vi "Read Date and Time.vi"(8 "error in (no error)":errorcluster, 11 "VISA resource name":refnum<visa-resource-name>) -> (0 "error out":errorcluster, 1 "Time":string, 2 "Date":string, 3 "VISA resource name out":refnum<visa-resource-name>)   [LabVIEW 2014, in "Fluke 190 Series II.lvlib"]
doc: "Returns the date and time setting of the real time clock in the testtool."
uses:
  Fluke 190 Series II.lvlib
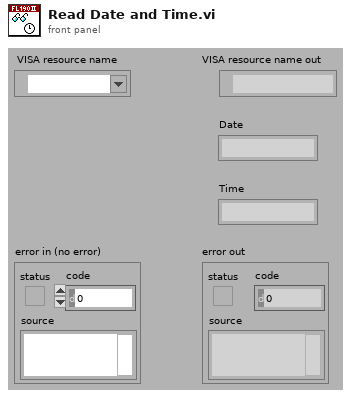
[diagram p1: front panel]
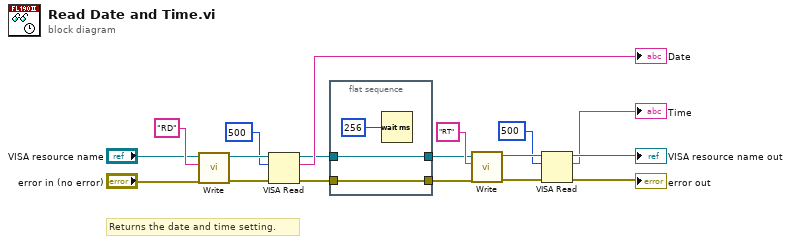
[diagram p0: block diagram]
diagram:
  # "Returns the date and time setting."
  n1 = call "Write.vi"("error in (no error)"="error in (no error)", "Write Buffer"="RD", "VISA resource name"="VISA resource name") -> ("error out"=w14:errorcluster, "VISA resource name out"=w15:refnum<visa-resource-name>)  [unwired: 7 out]
  n2 = VISA Read(VISA resource name=w15, byte count=u32 500, error in (no error)=w14) -> (VISA resource name out=w4:refnum<visa-resource-name>, read buffer=→"Date":string, error out=w2:errorcluster)  [unwired: 1 out]
  n3 = flat-sequence {
    tunnel: w4 -> [w21]
    tunnel: [w21] -> w3
    tunnel: w2 -> [w20]
    tunnel: [w20] -> w1
    frame #0 {
      n4 = Wait (ms)(milliseconds to wait=u32 256) -> ()  [unwired: 1 out]
    }
  }
  n5 = call "Write.vi"("error in (no error)"=w1, "Write Buffer"="RT", "VISA resource name"=w3) -> ("error out"=w11:errorcluster, "VISA resource name out"=w12:refnum<visa-resource-name>)  [unwired: 7 out]
  n6 = VISA Read(VISA resource name=w12, byte count=u32 500, error in (no error)=w11) -> (VISA resource name out=→"VISA resource name out":refnum<visa-resource-name>, read buffer=→"Time":string, error out=→"error out":errorcluster)  [unwired: 1 out]
